vi "JKI Parse State Queue with StateInfo.vi"(8 "error in (no error)":errorcluster, 11 "States Out":string) -> (1 "Arguments":string, 2 "Current State":string, 3 "Remaining States":string, 4 "String":string)   [LabVIEW 2014, in "FileSync -- Base.lvlib"]
uses:
  FileSync -- Base.lvlib
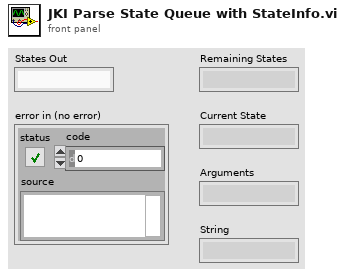
[diagram p1: front panel]
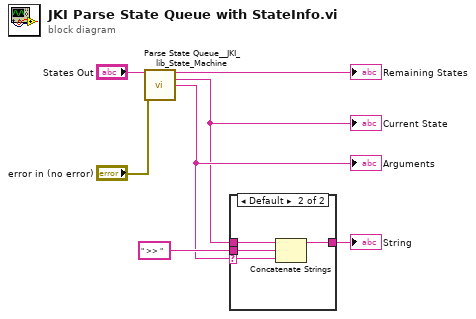
[diagram p0: block diagram]
diagram:
  n1 = call <vilib>:"Parse State Queue__JKI_lib_State_Machine.vi"("State Queue"="States Out", "Error In (no error)"="error in (no error)") -> ("Remaining States"=→"Remaining States":string, "Current State"=w4:string, "Arguments"=w6:string)  [unwired: 11 in]
  "Arguments" <- w6
  "Current State" <- w4
  n2 = case shown="Default" w6 {
    selector: w6 -> [_ w11]
    tunnel: " >> " ("string") -> [_ w12]
    tunnel: [w8 w10] -> w5
    tunnel: w4 -> [w8 w9]
    frame "" {
    }
    frame Default {
      n3 = Concatenate Strings(w9, w12, w11) -> (w10:string)
    }
  }
  "String" <- w5
